vi "Read_File_Sequencer.vi"(8 "error in (no error)":errorcluster caption="entrée d'erreur (pas d'erreur)", 11 "file path (dialog if empty)":path) -> (0 "error out":errorcluster caption="sortie d'erreur", 3 "Test Sequence":T1(array[cluster]))   [LabVIEW 2020, in "Library Commun.lvlib"]
uses:
  Library Commun.lvlib
  TypeDef/Type Function.ctl
  <vilib>/Utility/file.llb/Read Delimited Spreadsheet (string).vi
panel:
  out "Limit_Hight":string
  out "Limit_Low":string
  in  "Type Function":T2
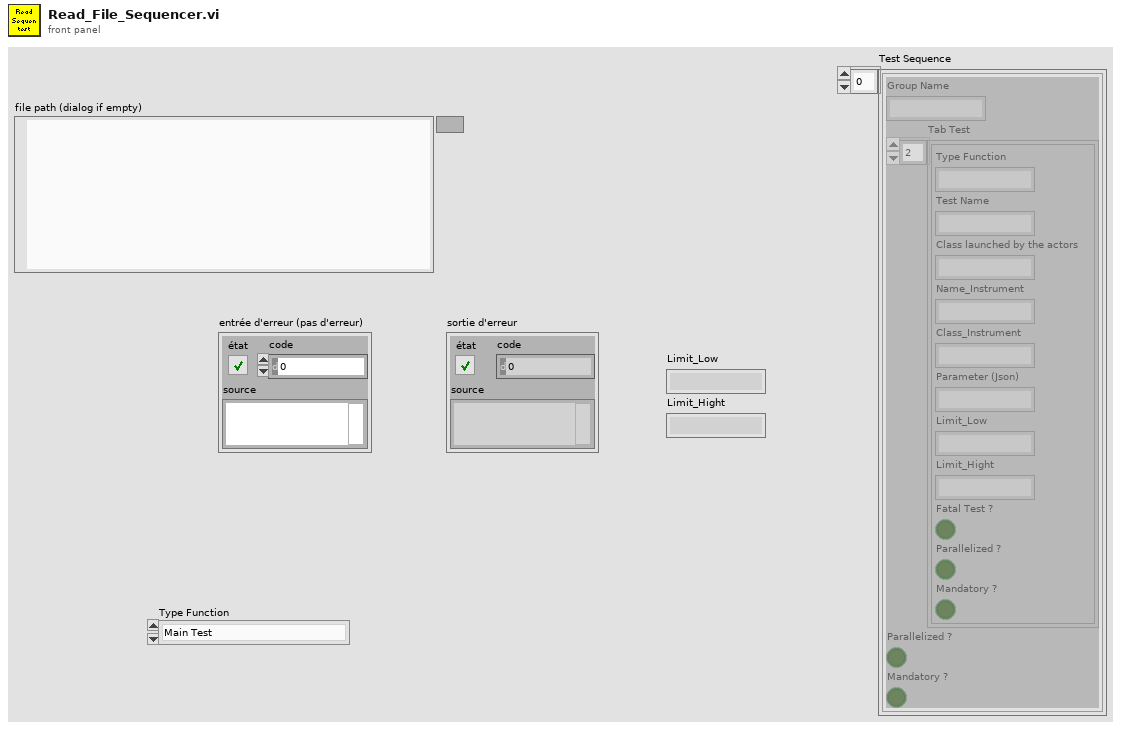
[diagram p1: front panel]
types:
  T1 = cluster{"Group Name":string, "Tab Test":cluster{"Type Function":string, "Test Name":string, "Class launched by the actors ":string, "Name_Instrument":string, "Class_Instrument":string, "Parameter (Json)":string, "Limit_Low":string, "Limit_Hight":string, "Fatal Test ?":bool, "Parallelized ?":bool, "Mandatory ?":bool}[], "Parallelized ?":bool, "Mandatory ?":bool}[]
  T2 = typedef "Library Commun.lvlib/Type Function.ctl" = enum16{"Main Test", "Function", "Thread", "Test"}
  T3 = cluster{"Group Name":string, "Tab Test":cluster{"Type Function":string, "Test Name":string, "Class launched by the actors ":string, "Name_Instrument":string, "Class_Instrument":string, "Parameter (Json)":string, "Limit_Low":string, "Limit_Hight":string, "Fatal Test ?":bool, "Parallelized ?":bool, "Mandatory ?":bool}[], "Parallelized ?":bool, "Mandatory ?":bool}
  T4 = cluster{"Type Function":string, "Test Name":string, "Class launched by the actors ":string, "Name_Instrument":string, "Class_Instrument":string, "Parameter (Json)":string, "Limit_Low":string, "Limit_Hight":string, "Fatal Test ?":bool, "Parallelized ?":bool, "Mandatory ?":bool}[]
  T5 = cluster{"Type Function":string, "Test Name":string, "Class launched by the actors ":string, "Name_Instrument":string, "Class_Instrument":string, "Parameter (Json)":string, "Limit_Low":string, "Limit_Hight":string, "Fatal Test ?":bool, "Parallelized ?":bool, "Mandatory ?":bool}
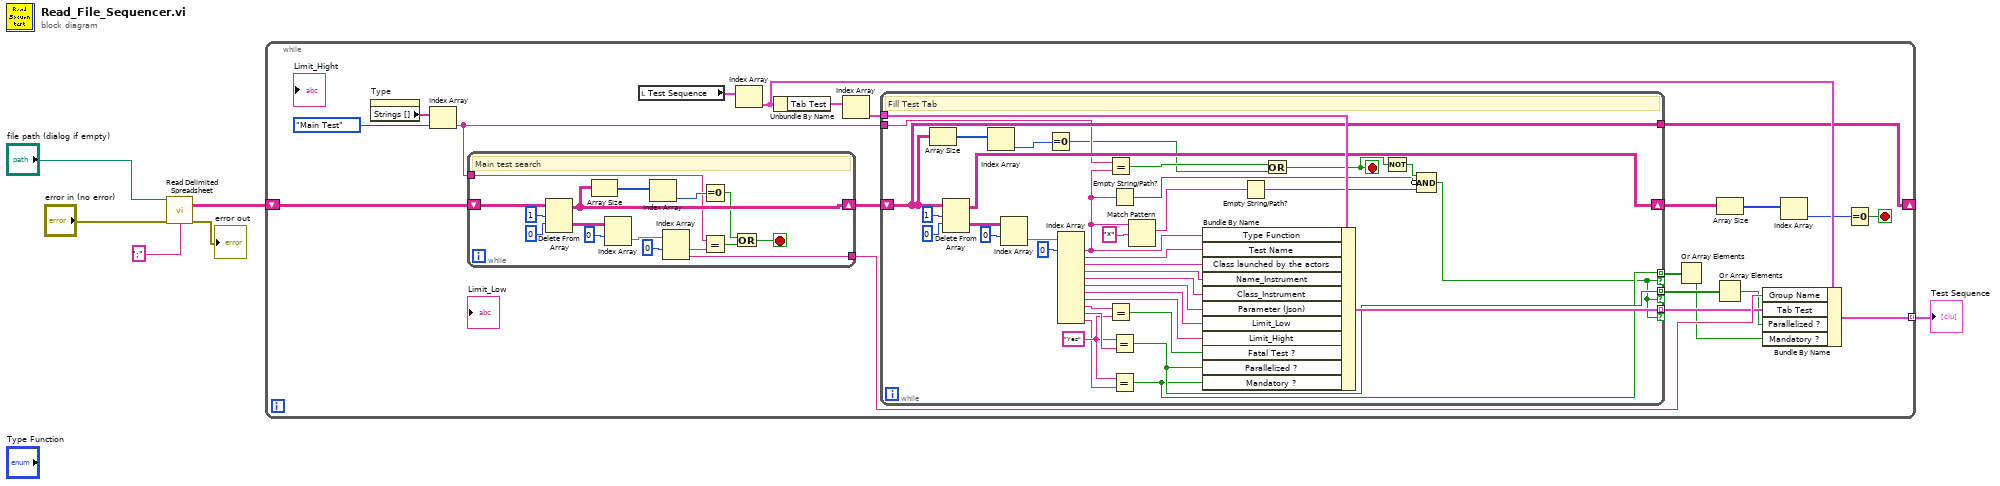
[diagram p0: block diagram]
diagram:
  n1 = call-poly <vilib>:"Read Delimited Spreadsheet.vi"("file path (dialog if empty)"="file path (dialog if empty)", "error in (no error)"="error in (no error)", "delimiter (\\t)"=";" ("delimiter (\\t)")) -> ("all rows"=w4:string[][], "error out"=→"error out":errorcluster)  [unwired: 7 in, 4 out]
  n2 = while {
    shift-right: [w18] -> _
    shift-left: w4 -> [w27]
    tunnel: [w15] -> w3 mode=indexing
    stop <- w11 stop-if-true
    n3 = property on="Type" class="Énum (strict)"() -> ("Strings []"=w20:string[])  [unwired: 2 in, 2 out]
    n4 = Index Array(array=w20, index=Type_Function."Main Test" ("Type")) -> (element=w17:string)
    n5 = while {
      shift-right: [w73] -> w25
      shift-left: w27 -> [w77]
      tunnel: [w69] -> w24
      tunnel: w17 -> [w68]
      stop <- w65 stop-if-true
      # "Main test search"
      n6 = Delete From Array(array=w77, length=1 ("longueur"), index (row)=0 ("indice (ligne)")) -> (deleted portion=w76:string[][], array with subset deleted=w73:string[][])  [unwired: 1 in]
      n7 = Array Size(array=w73) -> (size(s)=w72:i32[])
      n8 = Index Array(array=w76, index (row)=0 ("indice")) -> (element=w70:string[])  [unwired: 1 in]
      n9 = Index Array(array=w72) -> (element=w71:i32)  [unwired: 1 in]
      n10 = Index Array(array=w70, index #1=0 ("indice désactivé (col)")) -> (element #1=w75:string, element #2=w69:string)  [unwired: 1 in]
      n11 = Equal To 0?(x=w71) -> (x = 0?=w66:bool)
      n12 = Equal?(x=w68, y=w75) -> (x = y?=w67:bool)
      n13 = Or(x=w66, y=w67) -> (x .or. y?=w65:bool)
    }
    n14 = local read "Test Sequence"() -> (w26:T1)
    n15 = Index Array(array=w26) -> (element=w23:T3)  [unwired: 1 in]
    n16 = Unbundle By Name(w23) -> ("Tab Test"=w22:T4)
    n17 = Index Array(array=w22) -> (element=w21:T5)  [unwired: 1 in]
    n18 = while {
      shift-right: [w57] -> w13
      shift-left: w25 -> [w56]
      tunnel: w21 -> [w62]
      tunnel: [w56] -> w18
      tunnel: w17 -> [w55]
      tunnel: [w50] -> w16 mode=indexing if=w28
      tunnel: [w38] -> w10 mode=indexing if=w28
      tunnel: [w29] -> w8 mode=indexing if=w28
      stop <- w49 stop-if-true
      w31 = "Yes" ("y")
      # "Fill Test Tab"
      n19 = Array Size(array=w56) -> (size(s)=w64:i32[])
      n20 = Delete From Array(array=w56, length=1 ("longueur"), index (row)=0 ("indice (ligne)")) -> (deleted portion=w58:string[][], array with subset deleted=w57:string[][])  [unwired: 1 in]
      n21 = Index Array(array=w64) -> (element=w63:i32)  [unwired: 1 in]
      n22 = Index Array(array=w58, index (row)=0 ("indice")) -> (element=w51:string[])  [unwired: 1 in]
      n23 = Equal To 0?(x=w63) -> (x = 0?=w53:bool)
      n24 = Index Array(array=w51, index #1=0 ("indice désactivé (col)")) -> (element #1=w34:string, element #2=w48:string, element #3=w47:string, element #4=w46:string, element #5=w45:string, element #6=w37:string, element #7=w40:string, element #8=w39:string, element #9=w41:string, element #10=w42:string, element #11=w30:string)  [unwired: 10 in]
      n25 = Equal?(x=w55, y=w34) -> (x = y?=w54:bool)
      n26 = Equal?(x=w41, y=w31) -> (x = y?=w44:bool)
      n27 = Empty String/Path?(string/path=w34) -> (empty?=w33:bool)
      n28 = Equal?(x=w31, y=w42) -> (x = y?=w38:bool)
      n29 = Equal?(x=w31, y=w30) -> (x = y?=w29:bool)
      n30 = Match Pattern(string=w34, regular expression="*" ("chaîne recherchée")) -> (match substring=w35:string)  [unwired: 1 in, 3 out]
      n31 = Bundle By Name(cluster=w62, "Type Function"=w34, "Test Name"=w48, "Class launched by the actors"=w47, "Name_Instrument"=w46, "Class_Instrument"=w45, "Parameter (Json)"=w37, "Limit_Low"=w40, "Limit_Hight"=w39, "Fatal Test ?"=w44, "Parallelized ?"=w38, "Mandatory ?"=w29) -> (w50:T5)
      n32 = Empty String/Path?(string/path=w35) -> (empty?=w32:bool)
      n33 = Or(x=w54, y=w53) -> (x .or. y?=w49:bool)
      n34 = Not(x=w49) -> (.not. x?=w43:bool)
      n35 = Compound Arithmetic op=AND ("Opérateur arithmétique")(w43, invert w33, w32) -> (w28:bool)
    }
    n36 = Or Array Elements(Boolean array=w8) -> (logical OR=w7:bool)
    n37 = Or Array Elements(Boolean array=w10) -> (logical OR=w9:bool)
    n38 = Array Size(array=w13) -> (size(s)=w14:i32[])
    n39 = Bundle By Name(cluster=w23, "Group Name"=w24, "Tab Test"=w16, "Parallelized ?"=w9, "Mandatory ?"=w7) -> (w15:T3)
    n40 = Index Array(array=w14) -> (element=w12:i32)  [unwired: 1 in]
    n41 = Equal To 0?(x=w12) -> (x = 0?=w11:bool)
  }
  "Test Sequence" <- w3
